vi "harmonic_frequency.vi"(5 "FFT of FFT":dbl[][](array[numeric])) -> (0 "Fundamental Frequency":dbl, 1 "subarray":dbl[][](array[numeric]), 2 "XY Graph":cluster{"subarray":dbl[], "subarray":dbl[]}(graph), 4 "6*y":dbl)   [LabVIEW 2009]
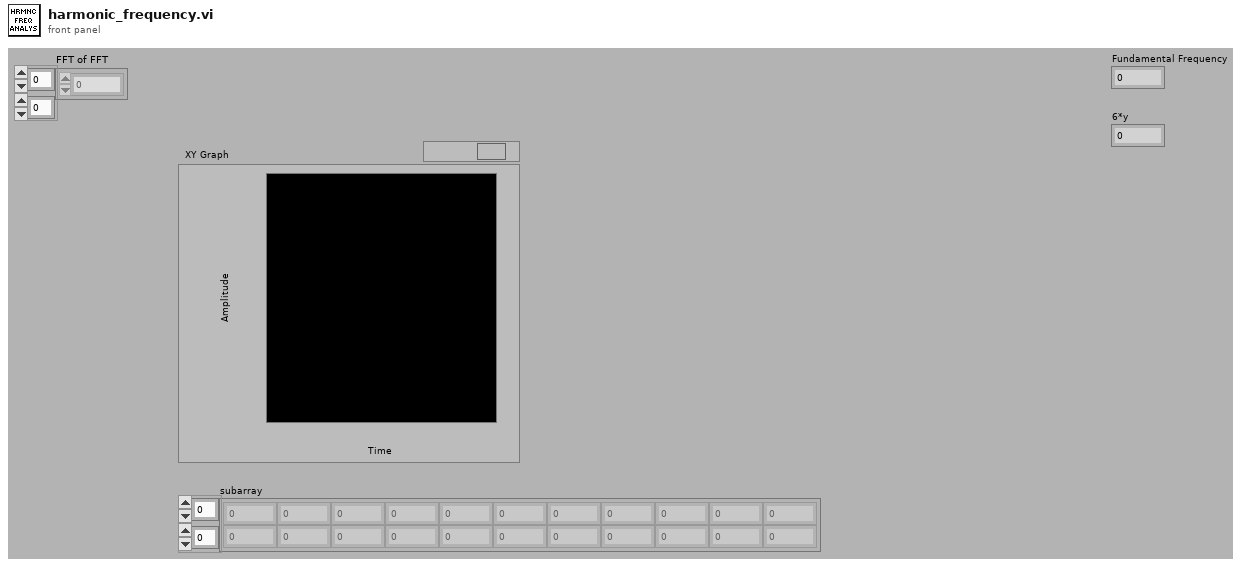
[diagram p1: front panel]
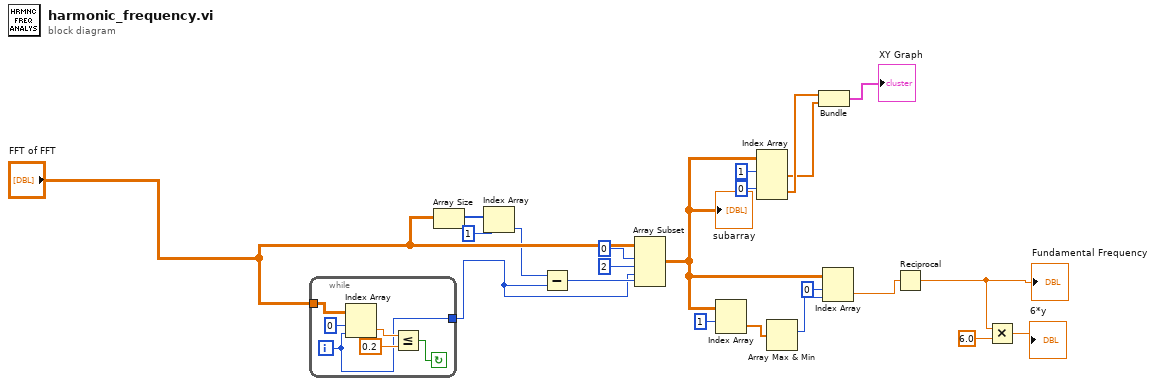
[diagram p0: block diagram]
diagram:
  n1 = while {
    tunnel: "FFT of FFT" -> [w28]
    tunnel: [w23] -> w12
    i -> [w23]
    stop <- w24 continue-if-true
    n2 = Index Array(array=w28, index (row)=0, index (col)=w23) -> (element=w26:dbl)
    n3 = Less Or Equal?(x=w26, y=0.2) -> (x <= y?=w24:bool)
  }
  n4 = Array Size(array="FFT of FFT") -> (size(s)=w6:i32[])
  n5 = Index Array(array=w6, index=1) -> (element=w8:i32)
  n6 = Subtract(x=w8, y=w12) -> (x-y=w13:i32)
  n7 = Array Subset(array="FFT of FFT", index (row)=0 ("index"), length (row)=2 ("length"), index (col)=w12, length (col)=w13) -> (w14:dbl[][])
  "subarray" <- w14
  n8 = Index Array(array=w14, index (row)=1) -> (element=w16:dbl[])  [unwired: 1 in]
  n9 = Index Array(array=w14, index (row) #1=1 ("index (row)"), index (row) #2=0 ("index (row)")) -> (element #1=w4:dbl[], element #2=w5:dbl[])  [unwired: 2 in]
  n10 = Array Max & Min(array=w16) -> (max index (indices)=w17:i32)  [unwired: 3 out]
  n11 = Bundle(w5, w4) -> (→"XY Graph":cluster{dbl[], dbl[]})  [unwired: 1 in]
  n12 = Index Array(array=w14, index (row)=0 ("disabled index (row)"), index (col)=w17) -> (element=w19:dbl)
  n13 = Reciprocal(x=w19) -> (1/x=w20:dbl)
  "Fundamental Frequency" <- w20
  n14 = Multiply(x=w20, y=6.0) -> (x*y=→"6*y":dbl)
